vi "test Fix Relocated Modules Updates Aliases.vi"(8 "error in (no error)":errorcluster, 11 "TestCase in":refnum<class "Routing and Faulting Scripting Unit Tests.lvclass">) -> (0 "error out":errorcluster, 3 "TestCase out":refnum<class "Routing and Faulting Scripting Unit Tests.lvclass">)   [LabVIEW 2017, in "Routing and Faulting Scripting Unit Tests.lvclass"]
uses:
  Routing and Faulting Scripting Unit Tests.lvclass
  Shared/VeriStand SLSC Scripting/Controls/SLSC Chassis ID.ctl
  Routing and Faulting Scripting Unit Tests.lvclass/Routing and Faulting Scripting Unit Tests.ctl
  NationalInstruments.VeriStand.SystemDefinitionAPI
  <vilib>/addons/_JKI Toolkits/VI Tester/TestCase.llb/TestCase.lvclass
  Routing and Faulting Scripting.lvlib
  Fake Hardware Custom Device/Fake Hardware Custom Device.lvlib
  Shared/VeriStand SLSC Scripting/VeriStand SLSC Scripting.lvlib
  Shared/Routing and Faulting Hardware API/Routing and Faulting Hardware API.lvlib
  C:/Program Files (x86)/National Instruments/LabVIEW 2017/vi.lib/addons/_JKI Toolkits/VI Tester/TestCase.llb/TestCase.lvclass
panel:
  in  "Save?":bool
  out "Output Filename":string
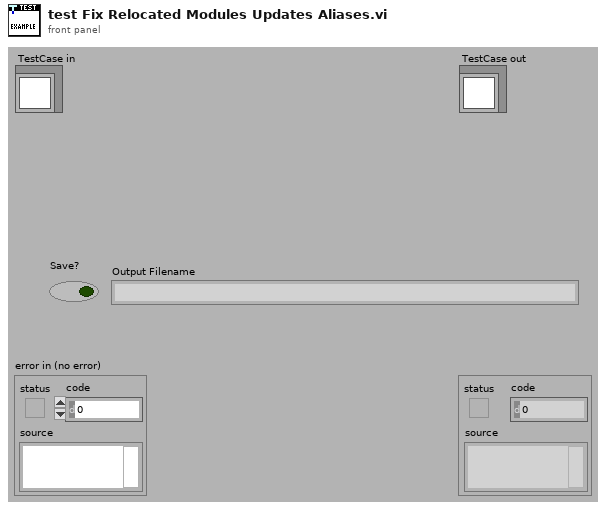
[diagram p1: front panel]
types:
  T1 = typedef "VeriStand SLSC Scripting.lvlib/SLSC Chassis ID.ctl" = cluster{"Name or IP":string, "ChassisIDType":i32, "chassisType":i32}
  T2 = typedef "Custom Device API.lvlib/Custom Device Item Ref.ctl" = u64
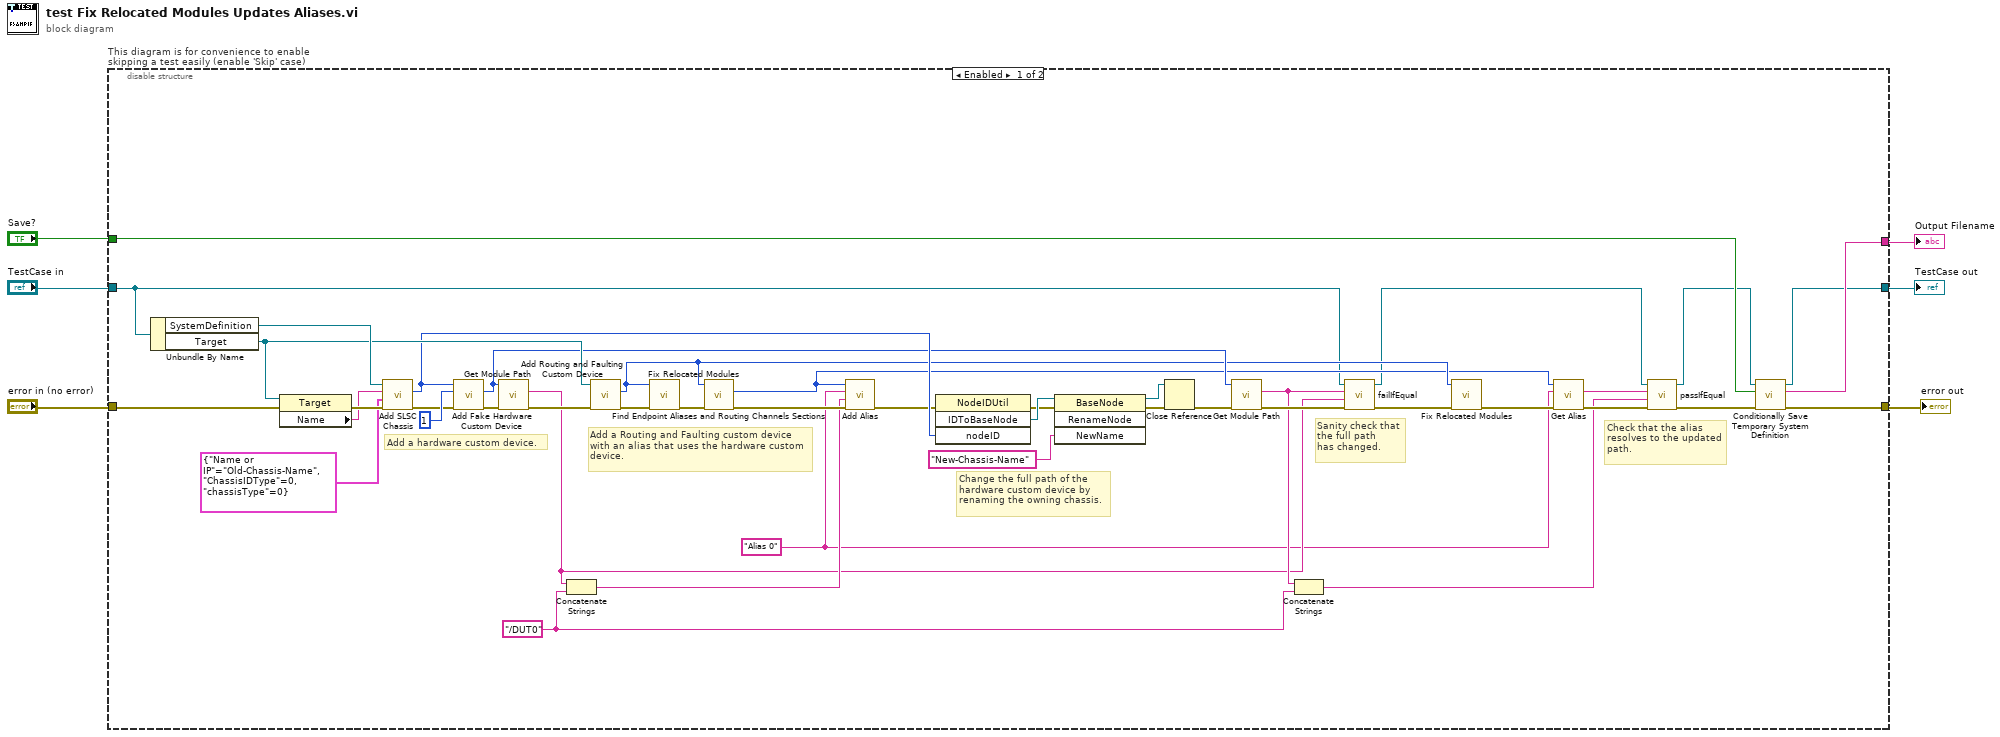
[diagram p0: block diagram]
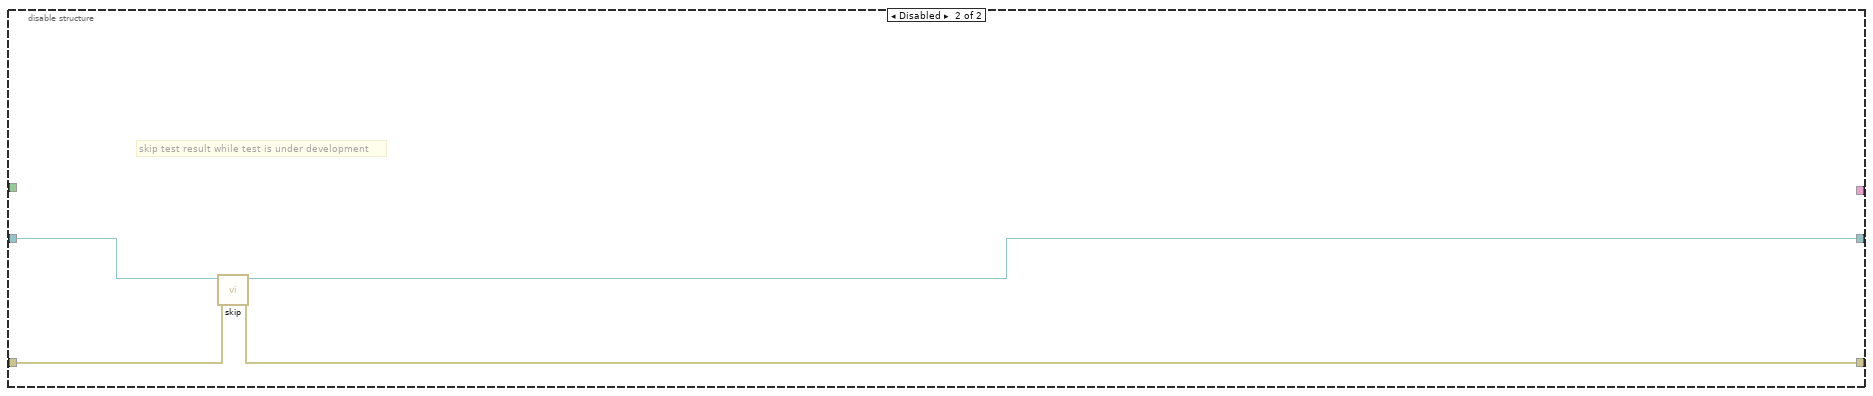
[diagram p2: hidden frame]
diagram:
  n1 = disable-structure "This diagram is for convenience to enable skipping a test easily (enable 'Skip' case)" shown="Enabled" {
    disable-tunnel: "TestCase in" -> [w12 w53]
    disable-tunnel: [w47 w51] -> w3
    disable-tunnel: [w48 w52] -> w5
    disable-tunnel: "error in (no error)" -> [w44 w50]
    disable-tunnel: [w49 _] -> w2
    disable-tunnel: "Save?" -> [w46 _]
    frame Enabled {
      w14 = "Alias 0" ("Alias")
      w21 = "/DUT0" ("string")
      # "Check that the alias\nresolves to the updated\npath."
      # "Sanity check that\nthe full path\nhas changed."
      # "Change the full path of the\nhardware custom device by\nrenaming the owning chassis."
      # "Add a Routing and Faulting custom device\nwith an alias that uses the hardware custom\ndevice."
      # "Add a hardware custom device."
      n2 = Unbundle By Name(w12) -> ("SystemDefinition"=w45:refnum<k24>, "Target"=w39:refnum<k24>)
      n3 = property class="Target"(reference=w39, error in=w44) -> (error out=w43:errorcluster, "Name"=w41:string)  [unwired: 1 out]
      n4 = call "Add SLSC Chassis.vi"("error in (no error)"=w43, "SLSC Chassis ID"=T1 {"Name or IP"="Old-Chassis-Name", "ChassisIDType"=0, "chassisType"=0}, "Target Name"=w41, "SysDef in"=w45) -> ("error out"=w34:errorcluster, "SLSC Chassis"=w26:u64)  [unwired: 5 in, 1 out]
      n5 = call "Add Fake Hardware Custom Device.vi"("error in (no error)"=w34, "Slot Number"=1, "SLSC Chassis Ref"=w26) -> ("error out"=w29:errorcluster, "Fake Hardware Custom Device Ref"=w24:T2)  [unwired: 6 in, 1 out]
      n6 = call "Get Module Path.vi"("error in (no error)"=w29, "Hardware Ref in"=w24) -> ("error out"=w28:errorcluster, "Resource"=w19:string)  [unwired: 6 in, 2 out]
      n7 = Concatenate Strings(w19, w21) -> (w27:string)
      n8 = call "Add Routing and Faulting Custom Device.vi"("error in (no error)"=w28, "Target in"=w39) -> ("error out"=w38:errorcluster, "Routing and Faulting Custom Device Ref"=w17:T2)  [unwired: 7 in, 1 out]
      n9 = call "Fix Relocated Modules.vi"("error in (no error)"=w38, "Routing and Faulting Ref in"=w17) -> ("error out"=w31:errorcluster)  [unwired: 8 in, 1 out]
      n10 = call "Find Endpoint Aliases and Routing Channels Sections.vi"("error in (no error)"=w31, "Routing and Faulting Custom Device Ref in"=w17) -> ("error out"=w30:errorcluster, "Endpoint Aliases Ref"=w16:T2)  [unwired: 6 in, 2 out]
      n11 = call "Add Alias.vi"("error in (no error)"=w30, "Endpoint"=w27, "Alias"=w14, "Endpoint Aliases Ref in"=w16) -> ("error out"=w25:errorcluster)  [unwired: 6 in, 1 out]
      n12 = invoke class="NodeIDUtil" method="IDToBaseNode"(error in=w25, "nodeID"=w26) -> (error out=w35:errorcluster, "IDToBaseNode"=w37:refnum<k24>)  [unwired: 2 in, 2 out]
      n13 = invoke class="BaseNode" method="RenameNode"(reference=w37, error in=w35, "NewName"="New-Chassis-Name") -> (reference out=w32:refnum<k24>, error out=w33:errorcluster)  [unwired: 1 in, 2 out]
      n14 = Close Reference(reference=w32, error in (no error)=w33) -> (error out=w23:errorcluster)
      n15 = call "Get Module Path.vi"("error in (no error)"=w23, "Hardware Ref in"=w24) -> ("error out"=w22:errorcluster, "Resource"=w20:string)  [unwired: 6 in, 2 out]
      n16 = Concatenate Strings(w20, w21) -> (w8:string)
      n17 = call-dynamic "failIfEqual.vi"("error in (no error)"=w22, "y"=w19, "x"=w20, "TestCase in"=w12) -> ("error out"=w18:errorcluster, "TestCase out"=w11:refnum<class "Routing and Faulting Scripting Unit Tests.lvclass">)  [unwired: 6 in]
      n18 = call "Fix Relocated Modules.vi"("error in (no error)"=w18, "Routing and Faulting Ref in"=w17) -> ("error out"=w15:errorcluster)  [unwired: 8 in, 1 out]
      n19 = call "Get Alias.vi"("error in (no error)"=w15, "Alias"=w14, "Endpoint Aliases Ref in"=w16) -> ("error out"=w13:errorcluster, "Endpoint"=w9:string)  [unwired: 6 in, 1 out]
      n20 = call-dynamic "passIfEqual.vi"("error in (no error)"=w13, "y"=w8, "x"=w9, "TestCase in"=w11) -> ("error out"=w7:errorcluster, "TestCase out"=w10:refnum<class "Routing and Faulting Scripting Unit Tests.lvclass">)  [unwired: 6 in]
      n21 = call "Conditionally Save Temporary System Definition.vi"("error in (no error)"=w7, "Save?"=w46, "Test Case"=w10) -> ("error out"=w48:errorcluster, "filename"=w49:string, "Test Case"=w47:refnum<class "Routing and Faulting Scripting Unit Tests.lvclass">)  [unwired: 6 in]
    }
    frame Disabled {
      # "skip test result while test is under development"
      n22 = call <vilib>:"skip.vi"("error in (no error)"=w50, "TestCase in"=w53) -> ("error out"=w52:errorcluster, "TestCase out"=w51:refnum<class "Routing and Faulting Scripting Unit Tests.lvclass">)  [unwired: 8 in]
    }
  }
  "error out" <- w5
  "TestCase out" <- w3
  "Output Filename" <- w2
